vi "DriveModuleControl_TUNE.vi"(4 "Time":dbl=-1.0 format="%33.4f", 6 "OutputsEnabled":bool, 8 "error in":errorcluster, 9 "Actual State":T1={"Speed"=0.0, "Angle"={"VALUE"=0.0, "COS"=1.0, "SIN"=0.0}} {"Angle"."SIN" format="%13.4f"; "Angle"."COS" format="%13.4f"; "Angle"."VALUE" format="%13.4f"}, 10 "Desired State":T1={"Speed"=0.0, "Angle"={"VALUE"=0.0, "COS"=1.0, "SIN"=0.0}} {"Angle"."SIN" format="%13.4f"; "Angle"."COS" format="%13.4f"; "Angle"."VALUE" format="%13.4f"}, 11 "ModualNamePrefix":i32) -> (0 "error out":errorcluster)   [LabVIEW 2023]
uses:
  <vilib>/Rock Robotics/WPI/ThirdParty/JAS_Junk/TrajLib/TypeDef/SWERVE_DRIVE_MODULE_STATE.ctl
  <vilib>/Rock Robotics/WPI/ThirdParty/JAS_Junk/TrajLib/TypeDef/ROTATION2D.ctl
  <vilib>/Rock Robotics/WPI/ThirdParty/JAS_Junk/TrajLib/SimpleMotorFF_Calculate.vi
  <vilib>/Rock Robotics/WPI/ThirdParty/JAS_Junk/TrajLib/PIDController_AtSetpoint.vi
  <vilib>/Rock Robotics/WPI/ThirdParty/JAS_Junk/TrajLib/PIDController_SetPIDF.vi
  <vilib>/Rock Robotics/WPI/ThirdParty/JAS_Junk/TrajLib/PIDController_SetDerivativeFilter.vi
  <vilib>/Rock Robotics/WPI/ThirdParty/JAS_Junk/TrajLib/PIDController_SetIntegratorRange.vi
  <vilib>/Rock Robotics/WPI/ThirdParty/JAS_Junk/TrajLib/PIDController_SetTolerancePandV.vi
  <vilib>/Rock Robotics/WPI/ThirdParty/JAS_Junk/TrajLib/PIDController_DisableContinousInput.vi
  <vilib>/Rock Robotics/WPI/ThirdParty/JAS_Junk/TrajLib/PIDController_EnableContinousInput.vi
  <vilib>/Rock Robotics/WPI/ThirdParty/JAS_Junk/TrajLib/PIDController_Reset.vi
  <vilib>/Rock Robotics/WPI/ThirdParty/JAS_Junk/TrajLib/PIDController_New.vi
  <vilib>/Rock Robotics/WPI/ThirdParty/JAS_Junk/TrajLib/PIDController_SetOutputLimits.vi
  <vilib>/Rock Robotics/WPI/ThirdParty/JAS_Junk/TrajLib/VI/PIDController_SetIntegratorZone.vi
  <vilib>/Rock Robotics/WPI/ThirdParty/JAS_Junk/TrajLib/SlewRateLimiter_New.vi
  <vilib>/Rock Robotics/WPI/ThirdParty/JAS_Junk/TrajLib/SlewRateLimiter_Reset.vi
  <vilib>/Rock Robotics/WPI/ThirdParty/JAS_Junk/TrajLib/SlewRateLimiter_Calculate.vi
  <vilib>/Rock Robotics/WPI/ThirdParty/JAS_Junk/TrajLib/SlewRateLimiter_SetRate.vi
  <vilib>/Rock Robotics/WPI/ThirdParty/JAS_Junk/TrajLib/LinearFilter_ResetToValue.vi
  <vilib>/Rock Robotics/WPI/ThirdParty/JAS_Junk/TrajLib/LinearFilter_Calculate.vi
  <vilib>/Rock Robotics/WPI/ThirdParty/JAS_Junk/TrajLib/PIDController_NewPeriod.vi
  <vilib>/Rock Robotics/WPI/ThirdParty/JAS_Junk/TrajLib/Util_GetTime.vi
  <vilib>/Rock Robotics/SystemInterfaces/NetworkCommunication/NetComm_UsageReport_report.vi
  <vilib>/Rock Robotics/WPI/ThirdParty/JAS_Junk/TrajLib/VI/Util_GetTime_U32.vi
  DriveGlobal.vi
  <vilib>/Rock Robotics/SystemInterfaces/Utilities/FPGA_UtilitiesRead LocalTime.vi
  <vilib>/Rock Robotics/WPI/ThirdParty/JAS_Junk/TrajLib/VI/Util_GetTime_U64.vi
  <vilib>/Rock Robotics/WPI/ThirdParty/Phoenix-LabVIEW/CANCoder/CTRE_Phoenix_CANcoder_RefNumRegistryGet.vi
  <vilib>/Rock Robotics/WPI/MotorControl/WPI_MotorControlRefNum Registry Get.vi
  <vilib>/Rock Robotics/Network Tables/NT Write Number.vi
  <vilib>/Rock Robotics/WPI/ThirdParty/JAS_Junk/TrajLib/Globals/Util_LibraryGlobals.vi
  <vilib>/Rock Robotics/WPI/ThirdParty/JAS_Junk/TrajLib/PIDController_AdvCalculate_FF_Sp_Pv.vi
  <vilib>/Rock Robotics/Network Tables/NT Write Integer.vi
  <vilib>/Rock Robotics/WPI/ThirdParty/JAS_Junk/TrajLib/LinearFilter_MovingAverage.vi
  <vilib>/Rock Robotics/WPI/ThirdParty/JAS_Junk/TrajLib/LinearFilter_LowPassBW1.vi
  <vilib>/Rock Robotics/WPI/ThirdParty/JAS_Junk/TrajLib/LinearFilter_LowPassBW2.vi
  <vilib>/Rock Robotics/WPI/ThirdParty/JAS_Junk/TrajLib/LinearFilter_HighPassBW1.vi
  <vilib>/Rock Robotics/WPI/ThirdParty/JAS_Junk/TrajLib/LinearFilter_HighPassBW2.vi
  <vilib>/Rock Robotics/Network Tables/NT Write Boolean.vi
  <vilib>/Rock Robotics/WPI/ThirdParty/JAS_Junk/TrajLib/Trajectory_Library.lvlib
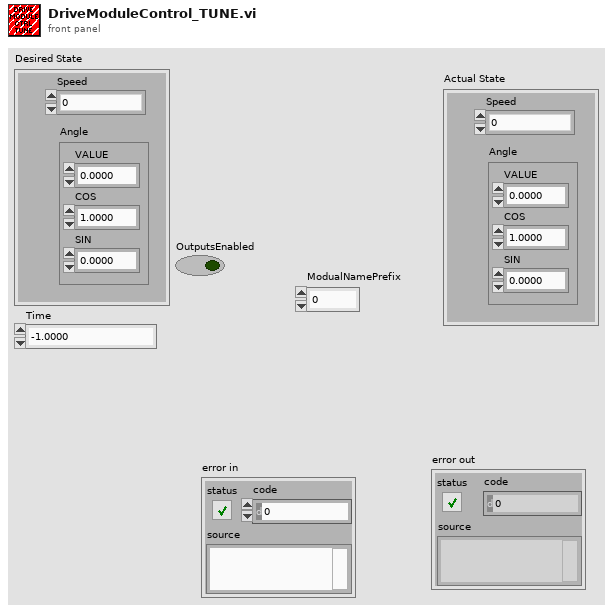
[diagram p1: front panel]
types:
  T1 = typedef "Trajectory_Library.lvlib/SWERVE_DRIVE_MODULE_STATE.ctl" = cluster{"Speed":dbl, "Angle":T2}
  T2 = typedef "Trajectory_Library.lvlib/ROTATION2D.ctl" = cluster{"VALUE":dbl, "COS":dbl, "SIN":dbl}
  T3 = enum16{"Ziegler Nicols - Fast", "Ziegler Nicols - Normal", "Ziegler Nicols - Slow", "CHR regulator - 0% overshoot", "CHR regulator - 20% overshoot", "CHR servo - 0 % overshoot", "CHR servo - 20% overshoot"}
  T4 = enum16{"Moving Average", "Low Pass 1st Order Butterworth", "Low Pass 2nd Order Butterworth", "High Pass 1st Order Butterworth", "High Pass 2nd Order Butterworth"}
  T5 = typedef "WPI_MotorControlDeviceRef.ctl" = cluster{"DeviceStatus":errorcluster, "Type":T6, "PWM":cluster{"PWM Channel":T7, "DeadBand":T8}, "CAN":cluster{"Device Number":u8, "SetOutput VI Ref":variant, "GetOutput VI Ref":variant, "Enable VI Ref":variant, "Disable VI Ref":variant, "Data":variant}, "Invert":bool, "DIO PWM":cluster{"PWM \"Enable\" Channel":T7, "DIOChannel":T9, "PWM Rate":dbl}}
  T6 = typedef "WPI_MotorControlType.ctl" = enum16{"PWM", "CAN", "DIO PWM"}
  T7 = typedef "FPGA_DIOPWMChannel.ctl" = enum8{"PWM 0", "PWM 1", "PWM 2", "PWM 3", "PWM 4", "PWM 5", "PWM 6", "PWM 7", "PWM 8", "PWM 9", "PWM MXP 0", "PWM MXP 1", "PWM MXP 2", "PWM MXP 3", "PWM MXP 4", "PWM MXP 5", "PWM MXP 6", "PWM MXP 7", "PWM MXP 8", "PWM MXP 9", "Invalid"}
  T8 = typedef "WPI_PWMDeadband.ctl" = cluster{"Name":string, "maxPositivePwm":i32, "minPositivePwm":i32, "centerPwm":i32, "maxNegativePwm":i32, "minNegativePwm":i32, "angularRange":u16}
  T9 = typedef "FPGA_DIOChannel.ctl" = enum8{"DIO 0", "DIO 1", "DIO 2", "DIO 3", "DIO 4", "DIO 5", "DIO 6", "DIO 7", "DIO 8", "DIO 9", "DIO MXP 0", "DIO MXP 1", "DIO MXP 2", "DIO MXP 3", "DIO MXP 4", "DIO MXP 5", "DIO MXP 6", "DIO MXP 7", "DIO MXP 8", "DIO MXP 9", "DIO MXP 10", "DIO MXP 11", "DIO MXP 12", "DIO MXP 13", "DIO MXP 14", "DIO MXP 15", "SPI Port CS1", "SPI Port CS2", "SPI Port CS3", "SPI Port MISO", "SPI Port MOSI", "Invalid"}
  T10 = typedef "Trajectory_Library.lvlib/SIMPLE_MOTOR_FF.ctl" = cluster{"Ks":dbl, "Kv":dbl, "Ka":dbl, "KnInv":dbl}
  T11 = typedef "Trajectory_Library.lvlib/PID_ADV_LIMITS.ctl" = cluster{"MaxInput":dbl, "MinInput":dbl, "Continuous":bool, "MaxOutput":dbl, "MinOutput":dbl}
  T12 = typedef "Trajectory_Library.lvlib/PID_ADV_TUNING.ctl" = cluster{"Kf":dbl, "Kp":dbl, "Ki":dbl, "Kd":dbl, "MaximumIntegral":dbl, "MinimumIntegral":dbl, "Filter Derivative":bool, "IntegralZone":dbl}
  T13 = cluster{"Controller Constant Type":enum16{"Ziegler Nicols - Fast", "Ziegler Nicols - Normal", "Ziegler Nicols - Slow", "CHR regulator - 0% overshoot", "CHR regulator - 20% overshoot", "CHR servo - 0 % overshoot", "CHR servo - 20% overshoot"}, "Type of Controller":enum16{"P", "PI", "PID"}, "CO Offset":dbl, "Kn":dbl, "Tuning Tolerance":dbl, "Plant Tolerance":dbl, "Newest Avg Time ":i32, "Long Ave Time":i32}
  T14 = cluster{"Plant Gain (K)":dbl, "Time Constant (T)":dbl, "Dead Time (L)":dbl, "stimulus operating point":dbl, "response operating point":dbl}
  T15 = cluster{"proportional gain (Kp)":dbl, "integral time (Ki / Sec)":dbl, "derivative time (Kd /Sec)":dbl}
  T16 = cluster{"Const Done":bool, "Plant Done":bool, "PV Std Dev":dbl, "CO Std Dev":dbl}
  T17 = typedef "Trajectory_Library.lvlib/SIMPLE_MOTOR_FF_KA_TUNE_PARAMS.ctl" = cluster{"Max SP":dbl, "Min Eval SP":dbl, "Max Eval SP":dbl, "Ramp Rate":dbl}
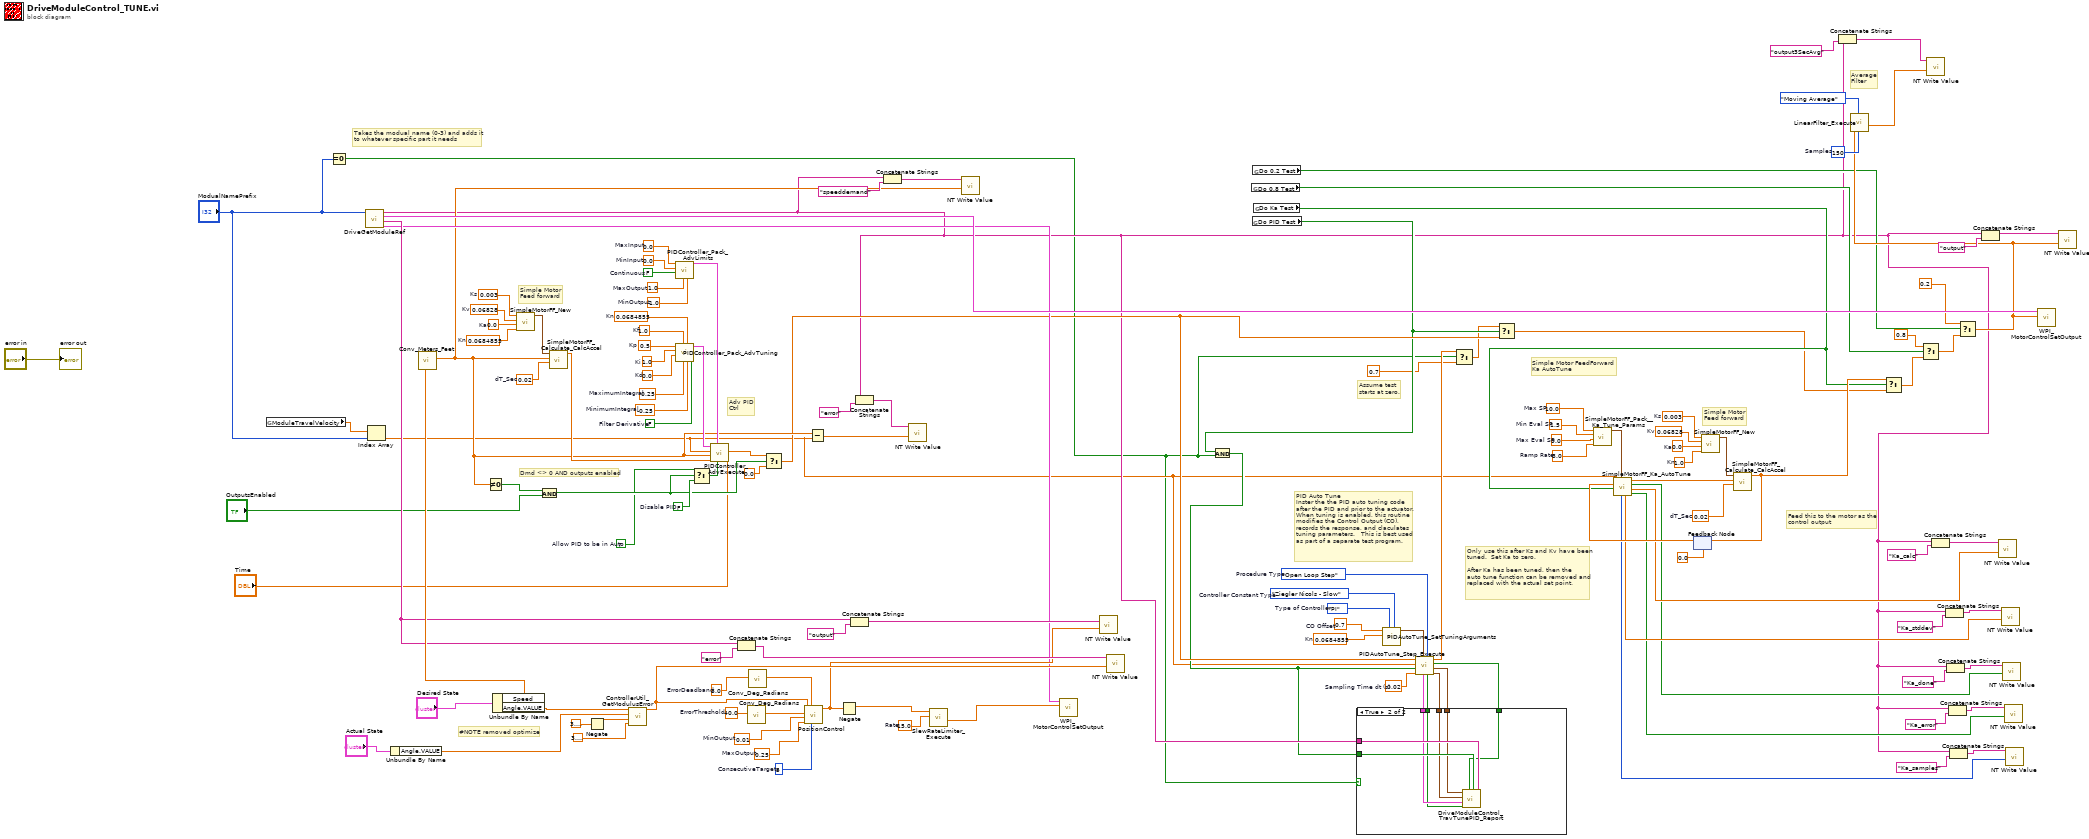
[diagram p0: block diagram]
diagram:
  w23 = 0.02  # Sampling Time dt (s)
  w22 = 0.0684855  # Kn
  w21 = 0.7  # CO Offset
  w20 = enum16{"P", "PI", "PID"}."PI"  # Type of Controller
  w19 = T3."Ziegler Nicols - Slow"  # Controller Constant Type
  w18 = enum16{"Open Loop Step", "Closed Loop Step"}."Open Loop Step"  # Procedure Type
  w54 = 1.0  # Kn
  w53 = 0.02  # dT_Sec
  w51 = 0.003  # Ks
  w50 = 0.06828  # Kv
  w49 = 0.0  # Ka
  w48 = 10.0  # Max SP
  w47 = 1.5  # Min Eval SP
  w46 = 9.0  # Max Eval SP
  w45 = 3.0  # Ramp Rate
  w65 = 150  # Samples
  w72 = 15.0  # Rate
  w73 = TRUE  # Allow PID to be in Auto
  w75 = FALSE  # Disable PID
  w84 = 0.0684855  # Kn
  w100 = 0.5  # Kp
  w99 = 1.0  # Ki
  w98 = 0.0  # Kd
  w97 = 1.0  # Kf
  w96 = 0.25  # MaximumIntegral
  w95 = -0.25  # MinimumIntegral
  w94 = FALSE  # Filter Derivative
  w92 = 0.0  # MinInput
  w91 = FALSE  # Continuous
  w90 = 1.0  # MaxOutput
  w93 = -1.0  # MinOutput
  w89 = 0.0  # MaxInput
  w109 = 0.0684855  # Kn
  w108 = 0.02  # dT_Sec
  w106 = 0.003  # Ks
  w105 = 0.06828  # Kv
  w104 = 0.0  # Ka
  w119 = 5  # ConsecutiveTargets
  w116 = 0.25  # MaxOutput
  w120 = 0.01  # MinOutput
  w113 = 40.0  # ErrorThreshold
  w115 = 3.0  # ErrorDeadband
  # "Assume test\nstarts at zero."
  # "PID Auto Tune\nInster the the PID auto tuning code\nafter the PID and prior to the actuator.\nWhen tuning is enabled, this routine\nmodifies the Control Output (CO), \nrecords the response, and claculates\ntuning parameters.   This is best used\nas part of a separate test program."
  # "Only use this after Ks and Kv have been\ntuned.  Set Ka to zero.\n\nAfter Ka has been tuned, then the \nauto tune function can be removed and\nreplaced with the actual set point."
  # "Feed this to the motor as the\ncontrol output"
  # "Simple Motor\nFeed forward"
  # "Simple Motor FeedForward\nKa AutoTune"
  # "Average\nFilter"
  # "#NOTE removed optimize"
  # "Dmd <> 0 AND outputs enabled"
  # "Adv PID\nCtrl"
  # "Simple Motor\nFeed forward"
  # "Takes the modual name (0-3) and adds it \nto whatever specific part it needs"
  n1 = global read "DriveGlobal.vi" "ModuleTravelVelocity"() -> (w85:dbl[])
  n2 = Equal To 0?(x="ModualNamePrefix") -> (x = 0?=w1:bool)
  n3 = call "DriveGetModuleRef.vi"("ModualNamePrefix"="ModualNamePrefix") -> ("SpinMot"=w101:T5, "SpinStr"=w102:string, "TravMot"=w103:T5, "TravStr"=w9:string)  [unwired: 5 in, 2 out]
  n4 = Index Array(array=w85, index="ModualNamePrefix") -> (element=w2:dbl)
  n5 = Unbundle By Name("Actual State") -> ("Angle.VALUE"=w123:dbl)
  n6 = Unbundle By Name("Desired State") -> ("Speed"=w110:dbl, "Angle.VALUE"=w124:dbl)
  n7 = call <vilib>:"Conv_Meters_Feet.vi"("Meters"=w110) -> ("Feet"=w80:dbl)  [unwired: 10 in]
  n8 = Not Equal To 0?(x=w80) -> (x != 0?=w77:bool)
  n9 = call <vilib>:"SimpleMotorFF_New.vi"("Kn"=w109, "Ka"=w104, "Kv"=w105, "Ks"=w106) -> ("SIMPLE_MOTOR_FF"=w107:T10)  [unwired: 7 in]
  n10 = And(x=w77, y="OutputsEnabled") -> (x .and. y?=w74:bool)
  n11 = call <vilib>:"SimpleMotorFF_Calculate_CalcAccel.vi"("dT_Sec"=w108, "VelSp"=w80, "SIMPLE_MOTOR_FF"=w107) -> ("FeedForward"=w86:dbl)  [unwired: 8 in]
  n12 = Negate(x=3.141592653589793) -> (-x=w125:dbl)
  n13 = call <vilib>:"ControllerUtil_GetModulusError.vi"("Maximum_Input"=3.141592653589793, "Minimum_Input"=w125, "Measurerment(PV)"=w123, "Reference(SP)"=w124) -> ("Error"=w117:dbl)  [unwired: 7 in]
  n14 = call <vilib>:"PIDController_Pack_AdvLimits.vi"("MinOutput"=w93, "MaxOutput"=w90, "Continuous"=w91, "MinInput"=w92, "MaxInput"=w89) -> ("Adv PID Limits"=w87:T11)  [unwired: 6 in]
  n15 = call <vilib>:"PIDController_Pack_AdvTuning.vi"("Filter Derivative"=w94, "MinimumIntegral"=w95, "Kn"=w84, "MaximumIntegral"=w96, "Kf"=w97, "Kd"=w98, "Ki"=w99, "Kp"=w100) -> ("Adv PID Tuning"=w88:T12)  [unwired: 3 in]
  n16 = Select(t=w73, s=w74, f=w75) -> (s? t:f=w76:bool)
  n17 = call <vilib>:"PIDController_AdvExecute.vi"("Time"="Time", "Auto"=w76, "Adv PID Limits"=w87, "FF-FeedForward"=w86, "SP-SetPoint"=w80, "PV-Measurement"=w2, "Adv PID Tuning"=w88) -> ("CO-ControlOutput"=w79:dbl)  [unwired: 2 in, 2 out]
  n18 = Concatenate Strings(w102, "error" ("refnum name")) -> (w128:string)
  n19 = call <vilib>:"Conv_Deg_Radians.vi"("Degress"=w113) -> ("Radians"=w112:dbl)  [unwired: 10 in]
  n20 = call <vilib>:"Conv_Deg_Radians.vi"("Degress"=w115) -> ("Radians"=w114:dbl)  [unwired: 10 in]
  n21 = Select(t=w79, s=w74, f=0.0 ("t")) -> (s? t:f=w16:dbl)
  n22 = call "PositionControl.vi"("ConsecutiveTargets"=w119, "ErrorDeadband"=w114, "MaxOutput"=w116, "MinOutput"=w120, "ErrorThreshold"=w112, "Error"=w117) -> ("OutputValue"=w111:dbl)  [unwired: 3 in, 2 out]
  n23 = Subtract(x=w80, y=w2) -> (x-y=w81:dbl)
  n24 = Negate(x=w111) -> (-x=w71:dbl)
  n25 = Concatenate Strings(w102, "output" ("refnum name")) -> (w118:string)
  n26 = Concatenate Strings(w9, "error" ("refnum name")) -> (w82:string)
  n27 = Concatenate Strings(w9, "speeddemand" ("refnum name")) -> (w132:string)
  n28 = call-poly <vilib>:"NT Write Value.vi"("value"=w81, "name"=w82) -> ()  [unwired: 9 in, 1 out]
  n29 = call <vilib>:"SlewRateLimiter_Execute.vi"("PositiveRate"=w72, "Input"=w71) -> ("Output"=w70:dbl)  [unwired: 8 in, 1 out]
  n30 = call-poly <vilib>:"NT Write Value.vi"("value"=w80, "name"=w132) -> ()  [unwired: 9 in, 1 out]
  n31 = call <vilib>:"WPI_MotorControlSetOutput.vi"("Output"=w70, "MotorControlDevRef"=w101) -> ()  [unwired: 7 in, 3 out]
  n32 = call-poly <vilib>:"NT Write Value.vi"("value"=w111, "name"=w118) -> ()  [unwired: 9 in, 1 out]
  n33 = call-poly <vilib>:"NT Write Value.vi"("value"=w117, "name"=w128) -> ()  [unwired: 9 in, 1 out]
  n34 = global read "DriveGlobal.vi" "Do 0.8 Test"() -> (w58:bool)
  n35 = global read "DriveGlobal.vi" "Do PID Test"() -> (w13:bool)
  n36 = And(x=w13, y=w1) -> (x .and. y?=w8:bool)
  n37 = global read "DriveGlobal.vi" "Do 0.2 Test"() -> (w59:bool)
  n38 = global read "DriveGlobal.vi" "Do Ka Test"() -> (w41:bool)
  n39 = call <vilib>:"PIDAutoTune_SetTuningArguments.vi"("Controller Constant Type"=w19, "Type of Controller"=w20, "Kn"=w22, "CO Offset"=w21) -> ("Configuration Parameters"=w17:T13)  [unwired: 7 in]
  n40 = call <vilib>:"PIDAutoTune_Step_Execute.vi"("Procedure Type"=w18, "Configuration Parameters"=w17, "Sampling Time dt (s)"=w23, "Tune"=w8, "Measurement  (PV)"=w2, "Control Output (Co)"=w16) -> ("Plant and Test Data"=w5:T14, "New Tuning Parameters"=w6:T15, "Tuning Done"=w7:bool, "Adj CO"=w12:dbl, "Error Occured"=w3:bool, "Diagnostic Info"=w4:T16)
  n41 = case shown="True" w1 {
    tunnel: w9 -> [_ w141]
    tunnel: w8 -> [_ w140]
    tunnel: w7 -> [_ w139]
    tunnel: w6 -> [_ w138]
    tunnel: w5 -> [_ w137]
    tunnel: w4 -> [_ w136]
    tunnel: w3 -> [_ w135]
    frame False {
    }
    frame True {
      n42 = call "DriveModuleControl_TravTunePID_Report.vi"("Network Table Prefix"=w141, "TestInProgress"=w140, "Tuning Done"=w139, "Error Occured"=w135, "Diagnostic Info"=w136, "Plant and Test Data"=w137, "New Tuning Parameters"=w138) -> ()  [unwired: 5 in]
    }
  }
  n43 = Select(t=w12, s=w1, f=0.7) -> (s? t:f=w11:dbl)
  n44 = Select(t=w11, s=w13, f=w16) -> (s? t:f=w15:dbl)
  n45 = call <vilib>:"SimpleMotorFF_Pack__Ka_Tune_Params.vi"("Ramp Rate"=w45, "Max Eval SP"=w46, "Min Eval SP"=w47, "Max SP"=w48) -> ("Packed Params"=w44:T17)  [unwired: 7 in]
  n46 = feedback #1(0.0 ("FeedForward")) -> (w56:dbl)
  n47 = call <vilib>:"SimpleMotorFF_Ka_AutoTune.vi"("SimpleMotorFeedforward_KaTune_Pack"=w44, "Run Test"=w41, "CO Control Output"=w56, "PV ProcessVariable"=w2) -> ("Error"=w26:bool, "Ka Calc"=w38:dbl, "Test Complete"=w32:bool, "SP Setpoint"=w55:dbl, "Ka StdDev"=w35:dbl, "Samples"=w29:i32)  [unwired: 1 in, 1 out]
  n48 = call <vilib>:"SimpleMotorFF_New.vi"("Kn"=w54, "Ka"=w49, "Kv"=w50, "Ks"=w51) -> ("SIMPLE_MOTOR_FF"=w52:T10)  [unwired: 7 in]
  n49 = call <vilib>:"SimpleMotorFF_Calculate_CalcAccel.vi"("dT_Sec"=w53, "VelSp"=w55, "SIMPLE_MOTOR_FF"=w52) -> ("FeedForward"=w42:dbl)  [unwired: 8 in]
  n50 = feedback-in #1(w42) -> ()
  n51 = Concatenate Strings(w9, "output3SecAvg" ("refnum name")) -> (w61:string)
  n52 = Select(t=w42, s=w41, f=w15) -> (s? t:f=w43:dbl)
  n53 = Select(t=0.8, s=w58, f=w43) -> (s? t:f=w66:dbl)
  n54 = Concatenate Strings(w9, "Ka_calc" ("refnum name")) -> (w39:string)
  n55 = Concatenate Strings(w9, "Ka_stddev" ("refnum name")) -> (w36:string)
  n56 = Concatenate Strings(w9, "Ka_done" ("refnum name")) -> (w33:string)
  n57 = Concatenate Strings(w9, "Ka_error" ("refnum name")) -> (w27:string)
  n58 = Concatenate Strings(w9, "Ka_samples" ("refnum name")) -> (w30:string)
  n59 = Select(t=0.2, s=w59, f=w66) -> (s? t:f=w63:dbl)
  n60 = call <vilib>:"LinearFilter_Execute.vi"("Samples"=w65, "Filter Type"=T4."Moving Average", "Input"=w63) -> ("Output"=w60:dbl)  [unwired: 7 in, 1 out]
  n61 = call-poly <vilib>:"NT Write Value.vi"("value"=w60, "name"=w61) -> ()  [unwired: 9 in, 1 out]
  n62 = Concatenate Strings(w9, "output" ("refnum name")) -> (w130:string)
  n63 = call-poly <vilib>:"NT Write Value.vi"("value"=w38, "name"=w39) -> ()  [unwired: 9 in, 1 out]
  n64 = call-poly <vilib>:"NT Write Value.vi"("value"=w35, "name"=w36) -> ()  [unwired: 9 in, 1 out]
  n65 = call-poly <vilib>:"NT Write Value.vi"("value"=w32, "name"=w33) -> ()  [unwired: 9 in, 1 out]
  n66 = call-poly <vilib>:"NT Write Value.vi"("value"=w26, "name"=w27) -> ()  [unwired: 9 in, 1 out]
  n67 = call-poly <vilib>:"NT Write Value.vi"("value"=w29, "name"=w30) -> ()  [unwired: 9 in, 1 out]
  n68 = call <vilib>:"WPI_MotorControlSetOutput.vi"("Output"=w63, "MotorControlDevRef"=w103) -> ()  [unwired: 7 in, 3 out]
  n69 = call-poly <vilib>:"NT Write Value.vi"("value"=w63, "name"=w130) -> ()  [unwired: 9 in, 1 out]
  "error out" <- "error in"
